vi "MethodNodeSetCtrlVal.vi"   [LabVIEW 2012]
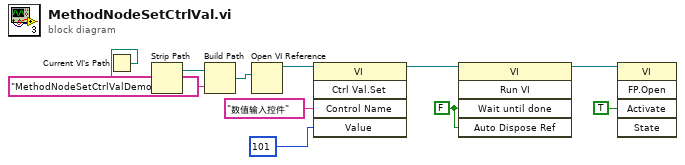
[diagram p0: block diagram]
diagram:
  w3 = FALSE ("结束前等待")
  n1 = Current VI's Path() -> (path=w11:path)
  n2 = Strip Path(path=w11) -> (stripped path=w10:path)  [unwired: 1 out]
  n3 = Build Path(base path=w10, name or relative path="MethodNodeSetCtrlValDemo.vi" ("名称或相对路径")) -> (appended path=w8:path)
  n4 = Open VI Reference(vi path=w8) -> (vi reference=w7:refnum<vi>)  [unwired: 5 in, 1 out]
  n5 = invoke class="VI" method="Ctrl Val.Set"(reference=w7, "Control Name"="数值输入控件" ("控件名"), "Value"=101) -> (reference out=w4:refnum<vi>)  [unwired: 2 in, 4 out]
  n6 = invoke class="VI" method="Run VI"(reference=w4, "Wait until done"=w3, "Auto Dispose Ref"=w3) -> (reference out=w2:refnum<vi>)  [unwired: 2 in, 4 out]
  n7 = invoke class="VI" method="FP.Open"(reference=w2, "Activate"=TRUE ("激活？")) -> ()  [unwired: 3 in, 5 out]
